vi "Handle NoTemplatesFound.vi"(8 "error in":errorcluster, 11 "GUI Objects":T1) -> (0 "error out":errorcluster)   [LabVIEW 2021]
doc: "Initialises or sets up the user-facing front panel (GUI) of the application.\nIncludes:\n1. Setting up the area of the front panel that is displayed to the user\n2. Opening or displaying the front panel"
uses:
  GUI Objects.ctl
  <vilib>/Utility/miscctls.llb/LVFontTypeDef.ctl
panel:
  # "Development\ncontrols/indicators useful for development and testing, but which are not outputs of the VI"
  # "Input\nInputs to the VI"
  # "Output\nOutputs of the VI"
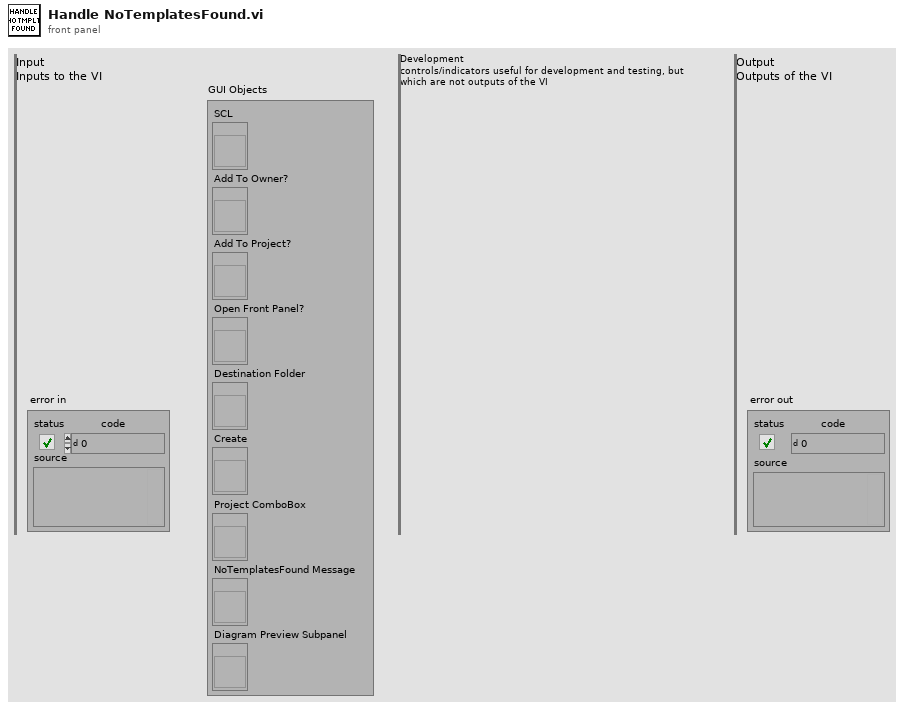
[diagram p1: front panel]
types:
  T1 = typedef "GUI Objects.ctl" = cluster{"SCL":refnum<vi>, "Add To Owner?":refnum<vi>, "Add To Project?":refnum<vi>, "Open Front Panel?":refnum<vi>, "Destination Folder":refnum<vi>, "Create":refnum<vi>, "Project ComboBox":refnum<vi>, "NoTemplatesFound Message":refnum<vi>, "Diagram Preview Subpanel":refnum<vi>}
  T2 = typedef "LVFontTypeDef.ctl" = cluster{"Font Name":string, "Size":u16, "Bold":bool, "Italic":bool, "Underline":bool, "Strikeout":bool, "Color":u32}
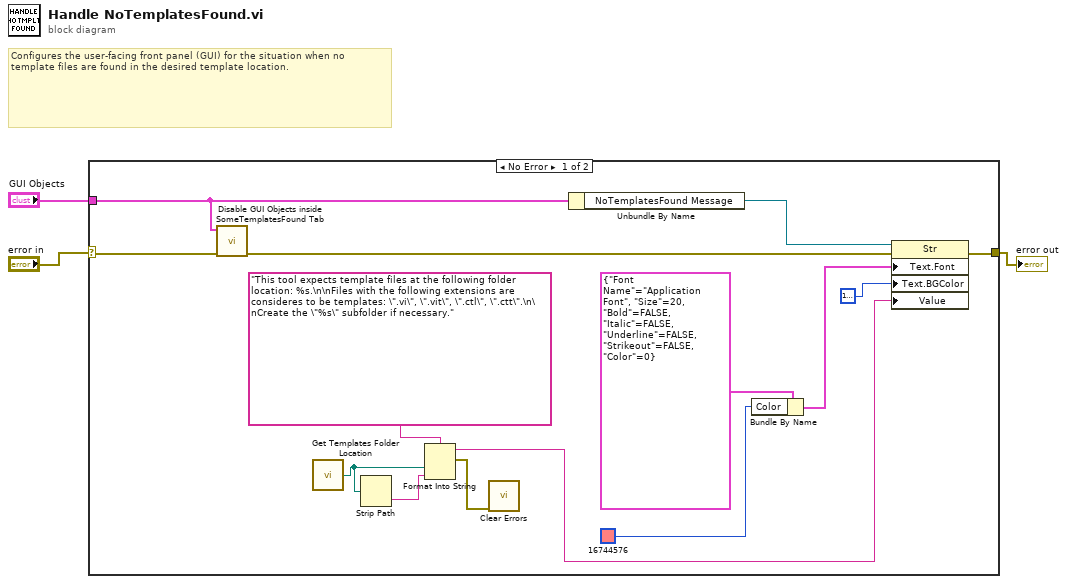
[diagram p0: block diagram]
diagram:
  # "Configures the user-facing front panel (GUI) for the situation when no template files are found in the desired template location."
  n1 = case shown="No Error" "error in" {
    selector: "error in" -> [w17 w18]
    tunnel: [w11 w18] -> w2
    tunnel: "GUI Objects" -> [w4 _]
    frame No Error {
      n2 = call "Disable GUI Objects inside SomeTemplatesFound Tab.vi"("error in"=w17, "GUI Objects"=w4) -> ("error out"=w5:errorcluster)  [unwired: 9 in]
      n3 = call "Get Templates Folder Location.vi"() -> ("Templates Folder Location"=w8:path)
      n4 = Strip Path(path=w8) -> (name=w7:string)  [unwired: 1 out]
      n5 = Format Into String(format string="This tool expects template files at the following folder location: %s.\n\nFiles with the following extensions are consideres to be templates: \".vi\", \".vit\", \".ctl\", \".ctt\".\n\nCreate the \"%s\" subfolder if necessary.", w8, w7) -> (resulting string=w6:string, error out=w9:errorcluster)  [unwired: 2 in]
      n6 = call <vilib>:"Clear Errors.vi"("error in (no error)"=w9) -> ()  [unwired: 5 in, 2 out]
      n7 = Unbundle By Name(w4) -> ("NoTemplatesFound Message"=w16:refnum<vi>)
      n8 = Bundle By Name(cluster=T2 {"Font Name"="Application Font", "Size"=20, "Bold"=FALSE, "Italic"=FALSE, "Underline"=FALSE, "Strikeout"=FALSE, "Color"=0} ("Text.Font"), "Color"=u32 16744576) -> (w13:T2)
      n9 = property class="Str"(reference=w16, error in=w5, "Text.Font"=w13, "Text.BGColor"=u32 16777216, "Value"=w6) -> (error out=w11:errorcluster)  [unwired: 1 out]
    }
    frame Error {
    }
  }
  "error out" <- w2
